vi "Main.vi"() -> ()   [LabVIEW 2017]
doc: "The myRIO Project template acquires acceleration data from the onboard accelerometer and displays the changes of acceleration values in a waveform chart."
uses:
  StateMachineControl.ctl
  <vilib>/Platform/TimedLoop/XDataNode/timing_clust.ctl
  <vilib>/Platform/TimedLoop/XDataNode/nitl_modes.ctl
  <vilib>/Platform/TimedLoop/XDataNode/wakeup.ctl
  <vilib>/myRIO/Instrument Drivers/Onboard IO/DIO/typedefs/DIO Reference.ctl
  <vilib>/myRIO/Common/Instrument Driver Framework/Utilities/typedefs/myRIO Generic Hardware Reference.ctl
  <vilib>/myRIO/Common/Instrument Driver Framework/Utilities/typedefs/Hardware Version Enum.ctl
  <vilib>/myRIO/Common/Instrument Driver Framework/Utilities/typedefs/myRIO v1.0 Reference.ctl
  <vilib>/myRIO/Common/Instrument Driver Framework/Utilities/typedefs/Generic FPGA Reference.ctl
  <vilib>/myRIO/Common/Instrument Driver Framework/myRIO v1.0/DIO/typedefs/DIO Channels List.ctl
  <vilib>/myRIO/Common/Instrument Driver Framework/myRIO v1.0/DIO/typedefs/DIO Channels Enum.ctl
  <vilib>/userdefined/High Color/nirio_resource_hc.ctl
  <vilib>/myRIO/Common/Instrument Driver Framework/myRIO v1.0/Encoder/typedefs/Encoder Signal Mode.ctl
  <vilib>/myRIO/Instrument Drivers/Onboard IO/Encoder/typedefs/Encoder Reference.ctl
  <vilib>/myRIO/Common/Instrument Driver Framework/myRIO v1.0/Encoder/typedefs/Encoder Channels Enum.ctl
  <vilib>/myRIO/Common/Instrument Driver Framework/myRIO v1.0/Encoder/typedefs/Encoder Configuration v1.0.ctl
  <vilib>/myRIO/Instrument Drivers/Onboard IO/PWM/typedefs/PWM Reference.ctl
  <vilib>/myRIO/Common/Instrument Driver Framework/myRIO v1.0/PWM/typedefs/PWM Channels Enum.ctl
  <vilib>/myRIO/Instrument Drivers/Onboard IO/PWM/typedefs/PWM Configuration.ctl
  <vilib>/myRIO/Common/Instrument Driver Framework/Utilities/vis/Is FPGA Ref Available.vi
  <vilib>/myRIO/Common/Instrument Driver Framework/myRIO v1.0/DIO/vis/myRIO v1.1 Open DIO.vi
  <vilib>/myRIO/Instrument Drivers/Onboard IO/DIO/vis/Read.vi
  <vilib>/myRIO/Instrument Drivers/Onboard IO/DIO/vis/Write.vi
  <vilib>/myRIO/Common/Instrument Driver Framework/myRIO v1.0/Encoder/vis/myRIO v1.1 Open Encoder.vi
  <vilib>/myRIO/Instrument Drivers/Onboard IO/Encoder/vis/Read.vi
  <vilib>/myRIO/Common/Instrument Driver Framework/myRIO v1.0/PWM/vis/myRIO v1.1 Open PWM.vi
  <vilib>/myRIO/Instrument Drivers/Onboard IO/PWM/vis/Set Duty Cycle and Frequency.vi
  <vilib>/myRIO/Common/Instrument Driver Framework/Utilities/vis/Validate Channels.vi
  <vilib>/myRIO/Common/Instrument Driver Framework/myRIO v1.0/DIO/vis/myRIO v1.0 Reserve DIO.vi
  <vilib>/myRIO/Common/Instrument Driver Framework/myRIO v1.0/Encoder/vis/myRIO v1.0 Reserve Encoder.vi
  <vilib>/myRIO/Common/Instrument Driver Framework/myRIO v1.0/PWM/vis/myRIO v1.0 Reserve PWM.vi
  <vilib>/myRIO/Common/Instrument Driver Framework/myRIO v1.0/UART/vis/myRIO v1.0 Close UART.vi
  <vilib>/myRIO/Common/Instrument Driver Framework/myRIO v1.0/Resource Manager/vis/myRIO v1.0 Reserve Channel List.vi
  <vilib>/myRIO/Common/Instrument Driver Framework/myRIO v1.0/DIO/vis/myRIO v1.0 Build MUX Configuration DIO.vi
  <vilib>/myRIO/Common/Instrument Driver Framework/myRIO v1.0/Encoder/vis/myRIO v1.0 Build MUX Configuration Encoder.vi
  <vilib>/myRIO/Common/Instrument Driver Framework/myRIO v1.0/PWM/vis/myRIO v1.0 Build MUX Configuration PWM.vi
  <vilib>/myRIO/Common/Instrument Driver Framework/myRIO v1.0/Resource Manager/vis/myRIO v1.0 Reserve Channel.vi
  <vilib>/myRIO/Common/Instrument Driver Framework/myRIO v1.0/Resource Manager/vis/myRIO v1.0 Unreserve Channel.vi
  <vilib>/myRIO/Common/Instrument Driver Framework/myRIO v1.0/Resource Manager/vis/myRIO v1.0 Create Configuration List.vi
  <vilib>/myRIO/Common/Instrument Driver Framework/myRIO v1.0/Resource Manager/vis/myRIO v1.0 Build Mutex Name.vi
  <vilib>/Utility/VariantDataType/GetNumericInfo.vi
  <vilib>/Utility/error.llb/Error Cluster From Error Code.vi
  <vilib>/myRIO/Common/Instrument Driver Framework/myRIO v1.0/myRIO v1.1 Open.vi
  <vilib>/myRIO/Common/Instrument Driver Framework/Utilities/vis/IO Manager.vi
  <vilib>/myRIO/Common/Instrument Driver Framework/Utilities/vis/Configuration Manager.vi
  <vilib>/myRIO/Common/Instrument Driver Framework/myRIO v1.0/Resource Manager/vis/myRIO v1.0 Configure IO.vi
  <vilib>/myRIO/Common/Instrument Driver Framework/myRIO v1.0/myRIO v1.0 Close.vi
  <vilib>/myRIO/Common/Instrument Driver Framework/myRIO v1.0/DIO/vis/myRIO v1.0 Read DIO.vi
  <vilib>/myRIO/Common/Instrument Driver Framework/myRIO v1.0/DIO/vis/myRIO v1.0 Write DIO.vi
  <vilib>/myRIO/Common/Instrument Driver Framework/myRIO v1.0/Encoder/vis/myRIO v1.0 Configure Encoder.vi
  <vilib>/myRIO/Common/Instrument Driver Framework/myRIO v1.0/Encoder/vis/myRIO v1.0 Read Encoder.vi
  <vilib>/myRIO/Common/Instrument Driver Framework/myRIO v1.0/PWM/vis/myRIO v1.0 Write PWM.vi
  <vilib>/myRIO/Common/Instrument Driver Framework/Utilities/vis/FPGA Ref Manager.vi
  <vilib>/myRIO/Common/Instrument Driver Framework/myRIO v1.0/myRIO v1.0 Reset FPGA.vi
  <vilib>/myRIO/Common/Instrument Driver Framework/myRIO v1.0/IRQ/vis/myRIO v1.0 IRQ Info FGV.vi
  <vilib>/myRIO/Common/Instrument Driver Framework/myRIO v1.0/IRQ/vis/myRIO v1.0 Timer IRQ Info FGV.vi
  <vilib>/myRIO/Common/Instrument Driver Framework/myRIO v1.0/IRQ/vis/myRIO v1.0 ISR Agent.vi
  <vilib>/Platform/TimedLoop/XDataNode/XDataNode.xnode
  <vilib>/myRIO/Express VI/Onboard Devices/Button/Button Express VI.xnode
  <vilib>/myRIO/Instrument Drivers/Onboard IO/DIO/vis/myRIO DIO Open.xnode
  <vilib>/myRIO/Express VI/Onboard Devices/LED/LED Express VI.xnode
  <vilib>/myRIO/Express VI/Onboard IO/Encoder/Encoder Express VI.xnode
  <vilib>/myRIO/Common/Instrument Driver Framework/myRIO v1.0/Encoder/typedefs/Encoder Count Direction Enum.ctl
  <vilib>/myRIO/Instrument Drivers/Onboard IO/Encoder/vis/myRIO Encoder Open.xnode
  <vilib>/myRIO/Express VI/Onboard IO/DO/DO Express VI.xnode
  <vilib>/myRIO/Express VI/Onboard IO/PWM/PWM Express VI.xnode
  <vilib>/myRIO/Instrument Drivers/Onboard IO/PWM/vis/myRIO PWM Open.xnode
  <vilib>/myRIO/Instrument Drivers/Utilities/Utilities.lvlib
  <vilib>/myRIO/Instrument Drivers/Onboard IO/Encoder/Encoder.lvlib
  <vilib>/myRIO/Instrument Drivers/Onboard IO/DIO/DIO.lvlib
  <vilib>/myRIO/Instrument Drivers/Onboard IO/PWM/PWM.lvlib
  <vilib>/Platform/TimedLoop/XDataNode/XDNodeRunTimeDep.lvlib
panel:
  in  "Marked Heading":dbl
  in  "Marked Distance":dbl
  in  "Go!":bool
  in  "Robot Heading":dbl
  out "Pixy Output Array":bool[](array[boolean])
  out "Detected":bool
  out "Data":string
  out "Color Signal Code":i32
  out "Object Actual Dist From Wall":dbl
  out "Object Y Average":dbl
  in  "Length":i32=90
  in  "Starting Index":i32
  out "Indexed Plot":cluster{dbl[], dbl[]}(graph)
  out "XY Graph":cluster{dbl[], dbl[]}(graph)
  in  "Robot Speed":dbl
  in  "Dist From Wall Setpoint":dbl=0.3
  out "LIDAR LOOP V_RIGHT":dbl
  out "LIDAR LOOP V_LEFT":dbl
  in  "Wall Tracking Boolean":bool
  out "Total Distance Travelled":dbl
  out "LIDAR Right x-avg (m)":dbl
  out "LIDAR Left x-avg (m)":dbl
  out "Min speed":dbl
  out "Max speed":dbl
  out "State":T1
  in  "Goal Position (m)":dbl[](array[numeric])=[2.0, 0.0]
  out "Theta Actual (rad)":dbl
  out "y":dbl
  out "x":dbl
  out "speed setpoint (m/s)":dbl
  out "chosen heading (rad)":dbl
  out "Output to PWM 2":dbl format="%.2f"
  out "Speed of Motor 2":dbl
  out "Motor 2 Total Distance":dbl
  out "Motor 2 Encoder Count":i32
  out "Counter Direction 2":enum16{"Counting Up", "Counting Down"}(ring)
  out "Overflow? 2":bool
  out "Motor 1 Total Distance":dbl
  out "Output to PWM":dbl format="%.2f"
  out "Speed of Motor 1":dbl
  out "Overflow?":bool
  out "Counter Direction":enum16{"Counting Up", "Counting Down"}(ring)
  out "Motor 1 Encoder Count":i32
  out "Error Out":errorcluster
  in  "Stop":bool
  # "Overview: This LabVIEW project is created to explore and analyse the data output provided by the encoder.\n\nAim of Encoder Data Analysis\n1. Process the number of counts generated by the encoder as the input.\n2. Output the motor speed and distance travelled."
  # "Motor 1"
  # "Motor 1 Encoder"
  # "Note: distance is in (m)"
  # "Note: speed is in (m/s)"
  # "Motor 2"
  # "Motor 2 Encoder"
  # "Note: speed is in (m/s)"
  # "Robot Control"
  # "Distance in m."
  # "Heading in (deg)."
  # "Speed is in m/s."
  # "Robot Position"
  # "Colour Sensor"
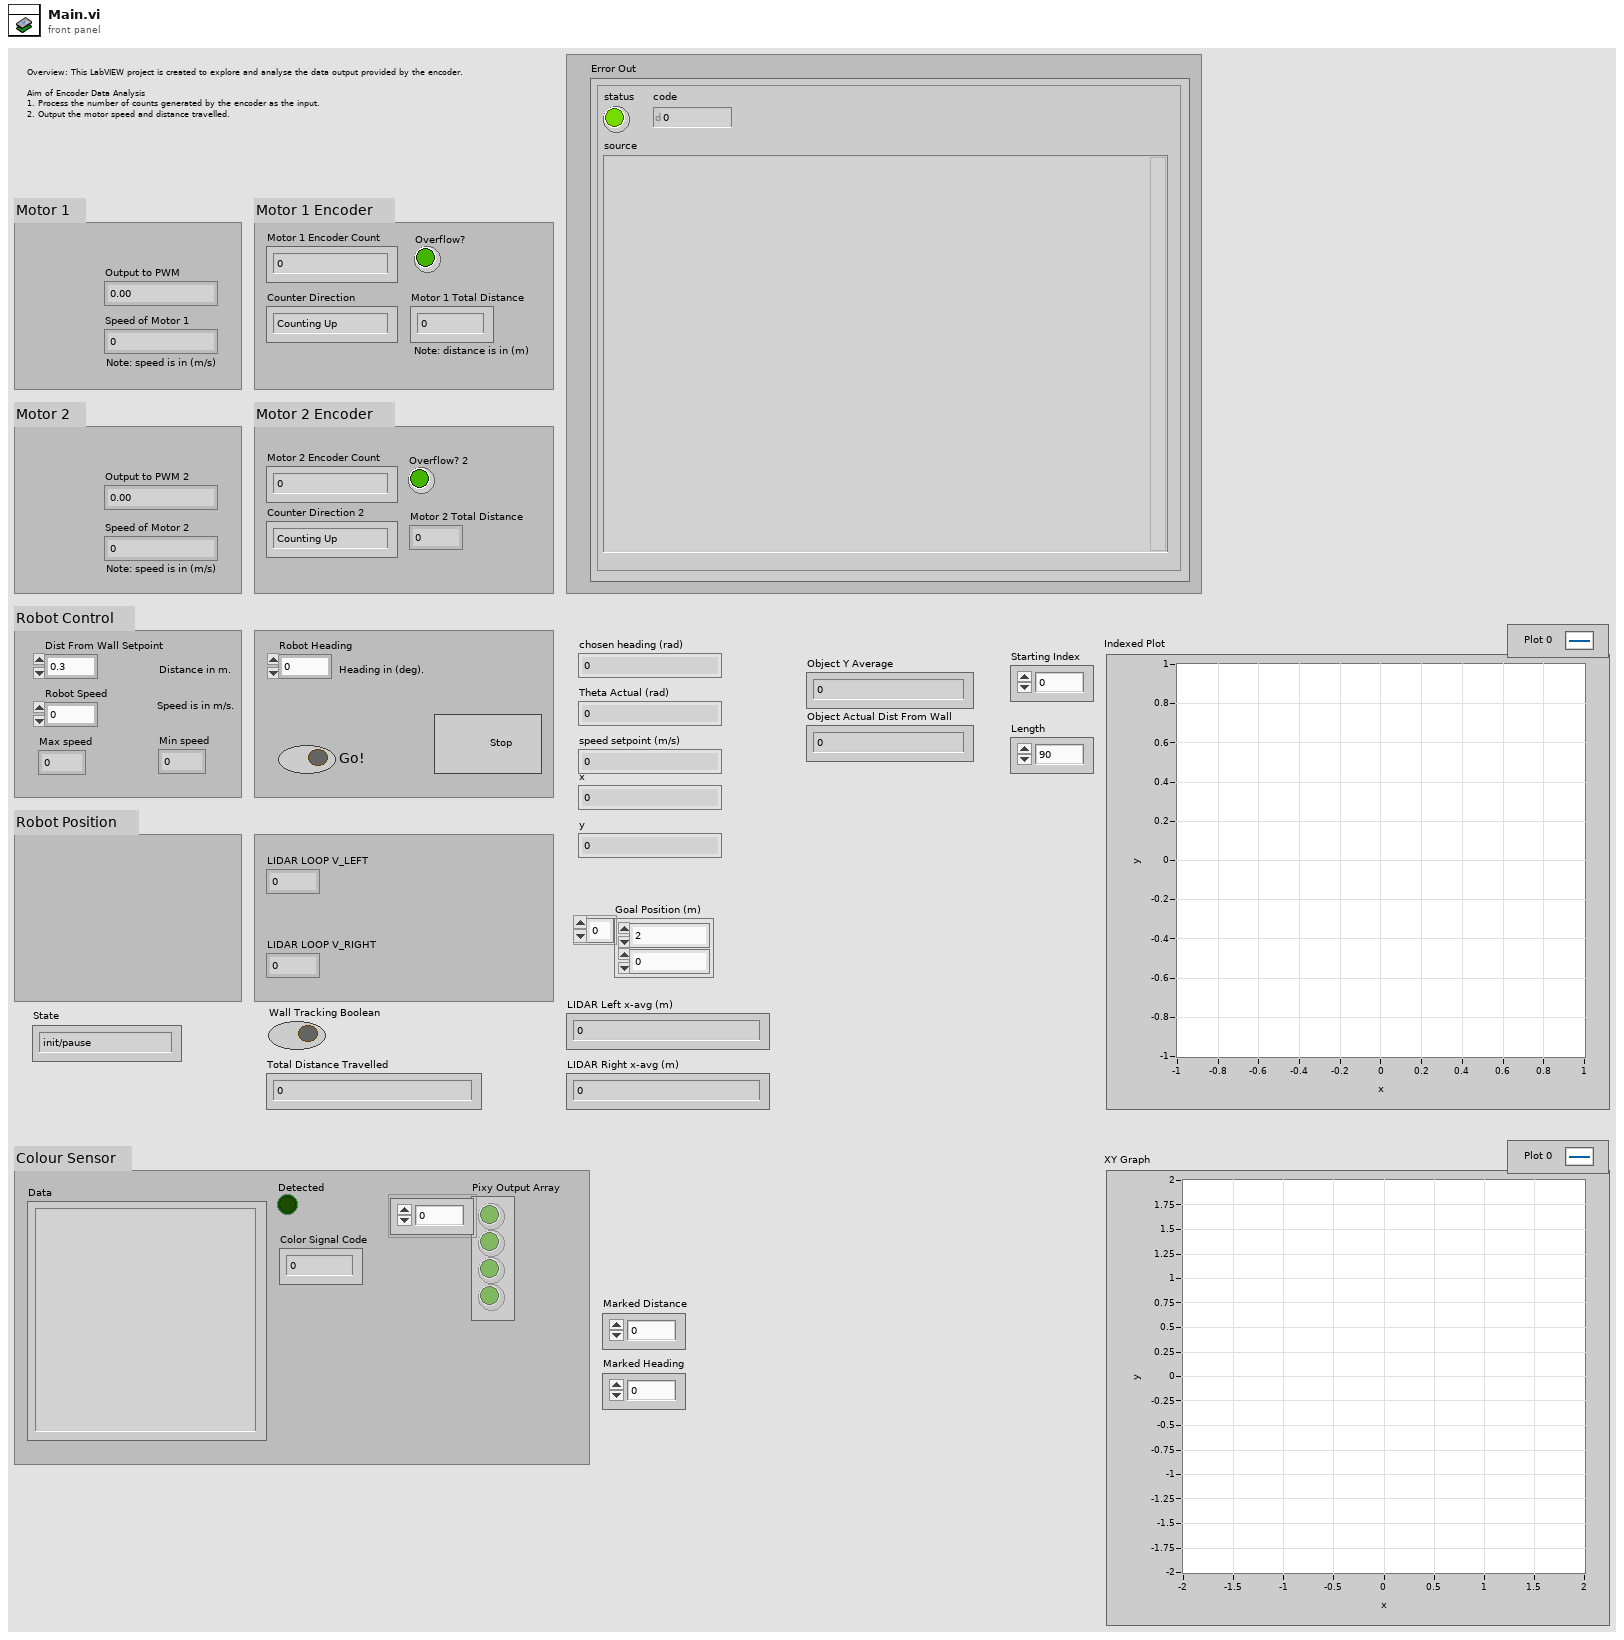
[diagram p1: front panel]
types:
  T1 = typedef "StateMachineControl.ctl" = enum16{"init/pause", "wall tracking w/ obs avoidance", "yellow zig-zag", "blue uneven surface", "red ramp", "green prepare to stop", "note down current distance", "go forward fixed dist & continue", "go forward fixed dist & stop", "stop finite state machine", "stop robot"}
  T2 = typedef "DIO.lvlib/DIO Reference.ctl" = cluster{"myRIO Reference":T3, "DIO Channels List":T7}
  T3 = typedef "myRIO Generic Hardware Reference.ctl" = cluster{"myRIO Model":T4, "myRIO Hardware Reference":T5}
  T4 = typedef "Hardware Version Enum.ctl" = enum16{"Unknown", "myRIO-1900", "myRIO-1950", "roboRIO", "NI ELVIS RIO CM"}
  T5 = typedef "myRIO v1.0 Reference.ctl" = cluster{"Generic FPGA Reference":T6, "Allow multiple opens":bool}
  T6 = typedef "Generic FPGA Reference.ctl" = refnum<k20>
  T7 = typedef "DIO Channels List.ctl" = T8[]
  T8 = typedef "DIO Channels Enum.ctl" = enum16{"Not Connected", "C/DIO0", "C/DIO1", "C/DIO2", "C/DIO3", "C/DIO4", "C/DIO5", "C/DIO6", "C/DIO7", "A/DIO0", "A/DIO1", "A/DIO2", "A/DIO3", "A/DIO4", "A/DIO5", "A/DIO6", "A/DIO7", "A/DIO8", "A/DIO9", "A/DIO10", "A/DIO11", "A/DIO12", "A/DIO13", "A/DIO14", "A/DIO15", "B/DIO0", "B/DIO1", "B/DIO2", "B/DIO3", "B/DIO4", "B/DIO5", "B/DIO6", "B/DIO7", "B/DIO8", "B/DIO9", "B/DIO10", "B/DIO11", "B/DIO12", "B/DIO13", "B/DIO14", "B/DIO15", "LED0", "LED1", "LED2", "LED3", "Button0", "DIO/DIO0", "DIO/DIO1", "DIO/DIO2", "DIO/DIO3", "DIO/DIO4", "DIO/DIO5", "DIO/DIO6", "DIO/DIO7", "DIO/DIO8", "DIO/DIO9", "SPI/CS0", "SPI/CS1", "SPI/CS2", "SPI/CS3", "LED RADIO (Green)", "LED RADIO (Red)", "LED COMM (Green)", "LED COMM (Red)", "LED MODE (Green)", "LED MODE (Red)"}
  T9 = typedef "nirio_resource_hc.ctl" = tag
  T10 = typedef "XDNodeRunTimeDep.lvlib/timing_clust.ctl" = cluster{"Expected End [f-1]":u64, "Actual End [f-1]":u64, "Finished Late? [f-1]":bool, "Expected End [i-1]":u64, "Actual End [i-1]":u64, "Finished Late? [i-1]":bool, "Expected Start [i]":u64, "Actual Start [i]":u64, "Expected Start [f]":u64, "Actual Start [f]":u64, "Source Name":string, "Structure Name":string, "Period":i64, "Deadline":i64, "Offset":i64, "Start":i64, "Priority":i32, "Timeout":i32, "Mode":T11, "Wakeup Reason":T12, "Error":errorcluster, "Source Type":string, "Secondary Source Type":string, "Global End Time":u64, "Global Start Time":u64, "Frame Duration":u64, "Iteration Duration":u64, "Assigned CPU":i32, "I/O Scan Engine Mode":u32}
  T11 = typedef "XDNodeRunTimeDep.lvlib/nitl_modes.ctl" = enum32{"No Change", "Process missed periods, maintain original phase", "Discard missed periods, maintain original phase", "Process missed periods, ignore original phase", "Discard missed periods, ignore original phase"}
  T12 = typedef "XDNodeRunTimeDep.lvlib/wakeup.ctl" = enum32{"Normal", "Aborted", "Asynchronous wakeup", "Timing source error", "Timed loop error", "Timeout"}
  T13 = typedef "PWM.lvlib/PWM Reference.ctl" = cluster{"myRIO Reference":T3, "PWM Channels Enum":T14, "PWM Configuration":T15}
  T14 = typedef "PWM Channels Enum.ctl" = enum16{"Not Connected", "C/PWM0", "C/PWM1", "A/PWM0", "A/PWM1", "A/PWM2", "B/PWM0", "B/PWM1", "B/PWM2", "PWM/PWM0", "PWM/PWM1", "PWM/PWM2", "PWM/PWM3", "PWM/PWM4", "PWM/PWM5", "PWM/PWM6", "PWM/PWM7", "PWM/PWM8", "PWM/PWM9"}
  T15 = typedef "PWM.lvlib/PWM Configuration.ctl" = cluster{"Frequency":dbl, "Duty Cycle":dbl}
  T16 = typedef "Encoder.lvlib/Encoder Reference.ctl" = cluster{"myRIO Reference":T3, "Encoder Channels Enum":T17}
  T17 = typedef "Encoder Channels Enum.ctl" = enum16{"Not Connected", "C/ENC0", "C/ENC1", "A/ENC", "B/ENC", "DIO/ENC0", "DIO/ENC1", "DIO/ENC2", "DIO/ENC3", "DIO/ENC4"}
  T18 = typedef "Encoder Signal Mode.ctl" = enum16{"Quadrature phase signal", "Step and direction signal"}
  T19 = typedef "Encoder Count Direction Enum.ctl" = enum16{"Counting Up", "Counting Down"}
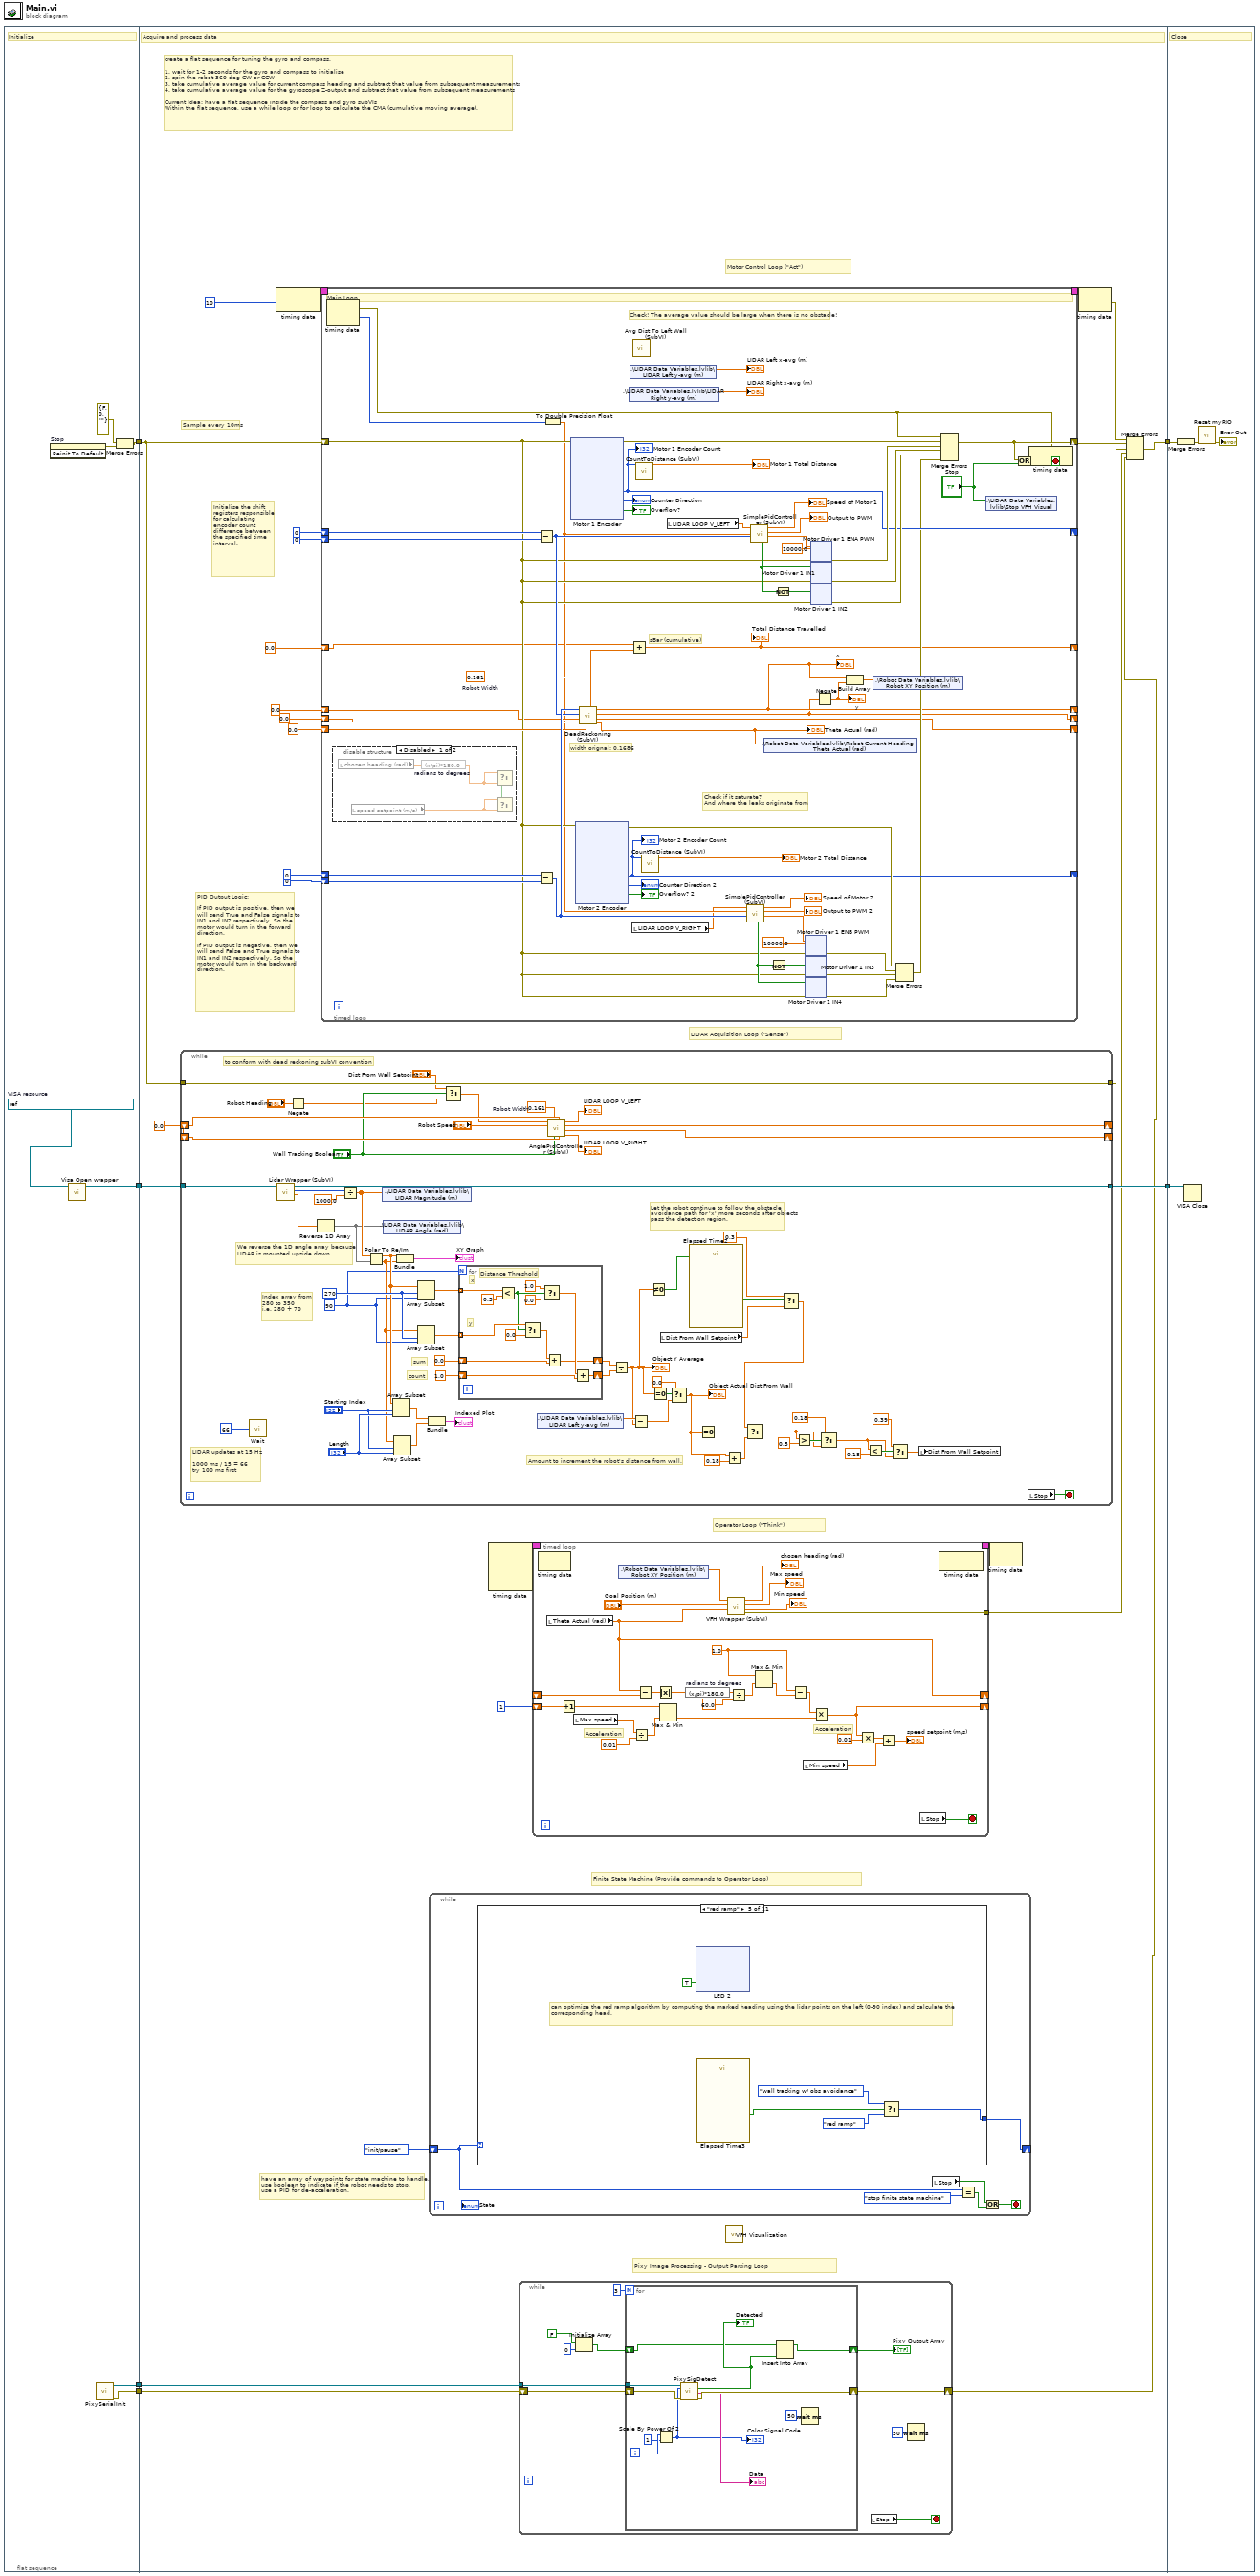
[diagram p0: block diagram]
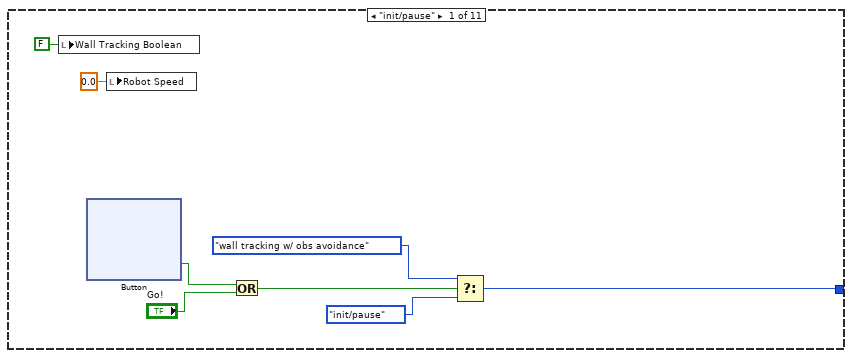
[diagram p2: hidden frame]
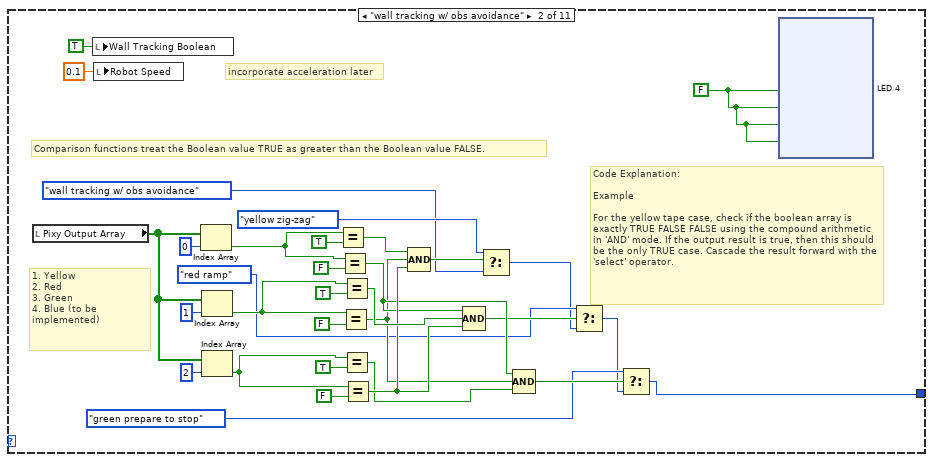
[diagram p3: hidden frame]
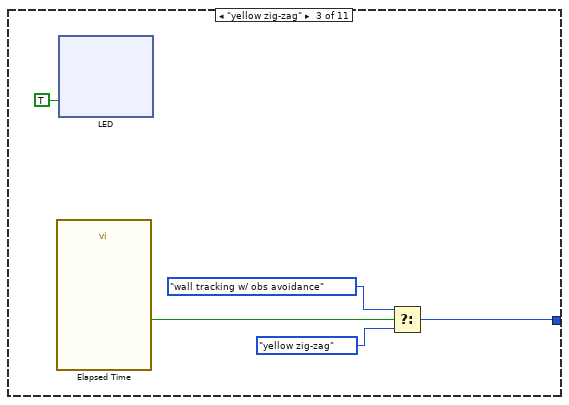
[diagram p4: hidden frame]
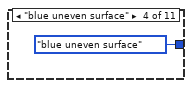
[diagram p5: hidden frame]
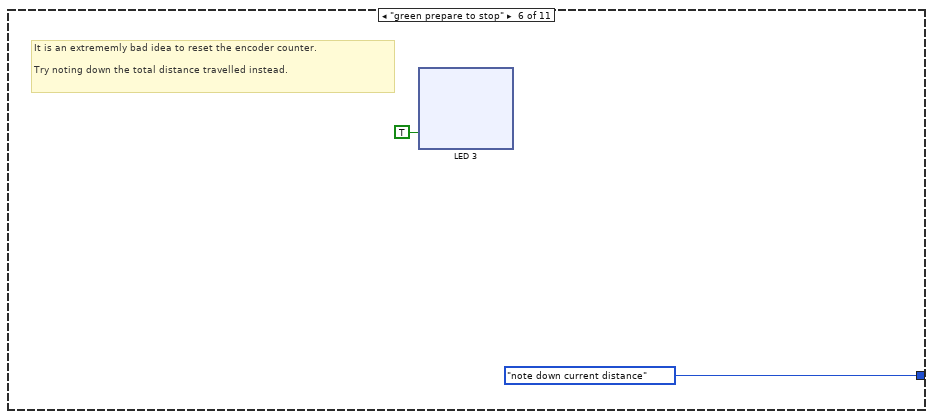
[diagram p6: hidden frame]
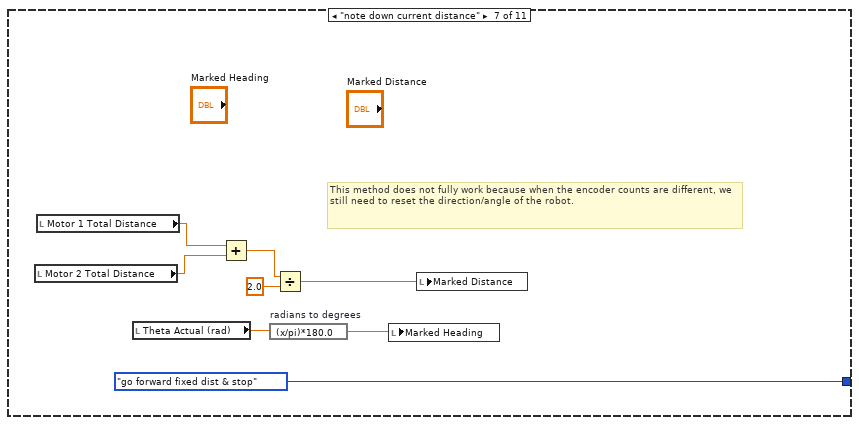
[diagram p7: hidden frame]
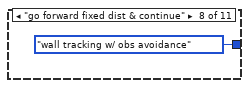
[diagram p8: hidden frame]
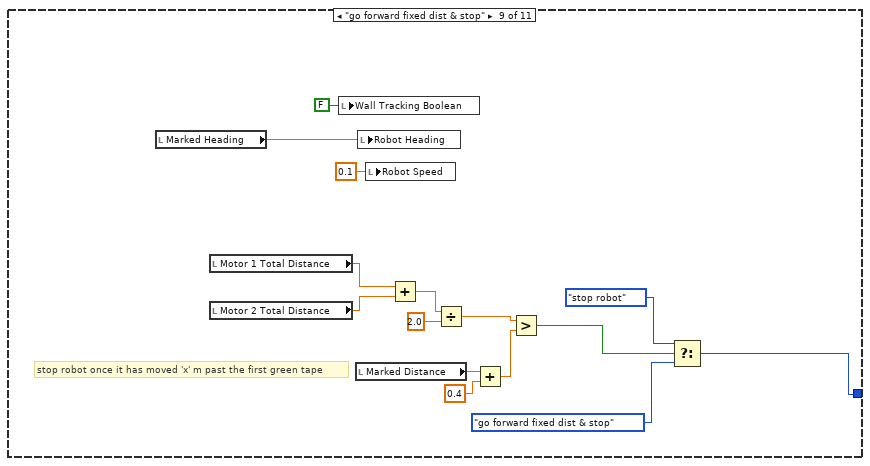
[diagram p9: hidden frame]
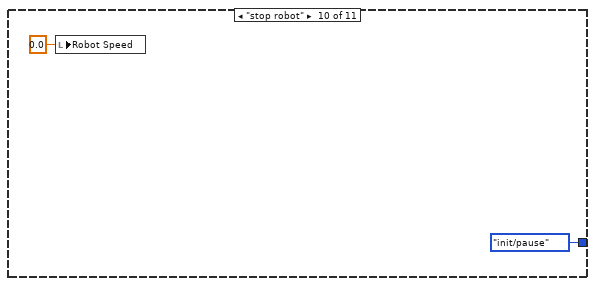
[diagram p10: hidden frame]
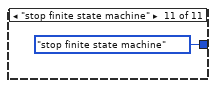
[diagram p11: hidden frame]
diagram:
  n1 = flat-sequence {
    tunnel: [w12] -> w6
    tunnel: [w10] -> w4
    tunnel: [w8] -> w2
    tunnel: [w7] -> w1
    tunnel: w6 -> [w26]
    tunnel: [w37] -> w5
    tunnel: w4 -> [w28]
    tunnel: [w27] -> w3
    tunnel: w2 -> [w16]
    tunnel: w1 -> [w15]
    tunnel: w5 -> [w810]
    tunnel: w3 -> [w811]
    frame #0 {
      w11 = refnum<visa-resource-name> "TCPIP::169.254.233.170::2112::SOCKET"  # VISA resource
      # "Initialize"
      n2 = invoke on="Stop" class="Bool (strict)" method="Reinit To Default"() -> (error out=w9:errorcluster)  [unwired: 3 in, 2 out]
      n3 = call "Visa Open wrapper.vi"("VISA resource"=w11) -> ("VISA resource name out"=w10:refnum<visa-resource-name>)  [unwired: 10 in]
      n4 = call "PixySerialInit.vi"() -> ("error out"=w7:errorcluster, "VISA resource name out"=w8:refnum<visa-resource-name>)  [unwired: 10 in]
      n5 = Merge Errors(errorcluster {"status"=FALSE, "code"=0, "source"=""} ("error in (no error)"), w9) -> (w12:errorcluster)
    }
    frame #1 {
      w18 = 0.0 ("Current Error")
      # "Pixy Image Processing - Output Parsing Loop"
      # "Finite State Machine (Provide commands to Operator Loop)"
      # "create a flat sequence for tuning the gyro and compass.\n\n1. wait for 1-2 seconds for the gyro and compass to initialise\n2. spin the robot 360 deg CW or CCW\n3. take cumulative average value for current compass heading and subtract that value from subsequent measurements\n4. take cumulative average value for the gyroscope Z-output and subtract that value from subsequent measurements\n\nCurrent Idea: have a flat sequence inside the compass and gyro subVIs\nWithin the flat sequence, use a while loop or for loop to calculate the CMA (cumulative moving average)."
      # "have an array of waypoints for state machine to handle,\nuse boolean to indicate if the robot needs to stop,\nuse a PID for de-acceleration."
      # "Operator Loop (\"Think\")"
      # "LIDAR Acquisition Loop (\"Sense\")"
      # "Motor Control Loop (\"Act\")"
      # "PID Output Logic:\n\nIf PID output is positive, then we will send True and False signals to IN1 and IN2 respectively. So the motor would turn in the forward direction.\n\nIf PID output is negative, then we will send False and True signals to IN1 and IN2 respectively. So the motor would turn in the backward direction."
      # "Initialise the shift registers responsible for calculating encoder count difference between the specified time interval."
      # "Sample every 10ms"
      # "Acquire and process data"
      n6 = while {
        tunnel: w28 -> [w419]
        tunnel: [w418] -> w27
        tunnel: w26 -> [w414]
        tunnel: [w414] -> w25
        shift-right: [w413] -> _
        shift-left: w18 -> [w411]
        shift-right: [w412] -> _
        shift-left: w18 -> [w410]
        stop <- w415 stop-if-true
        w392 = 90 ("length")
        w395 = 270 ("index")
        w407 = 0.161  # Robot Width
        # "to conform with dead reckoning subVI convention"
        # "Let the robot continue to follow the obstacle avoidance path for 'x' more seconds after objects pass the detection region."
        # "Amount to increment the robot's distance from wall."
        # "count"
        # "sum"
        # "Index array from 280 to 350\ni.e. 280 + 70"
        # "We reverse the 1D angle array because LIDAR is mounted upside down."
        # "LIDAR updates at 15 Hz\n\n1000 ms / 15 = 66\ntry 100 ms first"
        n7 = call "Wait"("Count(mSec)"=u32 66) -> ()  [unwired: 1 out]
        n8 = call "Lidar Wrapper (SubVI).vi"("VISA Refnum in"=w419) -> ("Array"=w401:dbl[], "Distance Array"=w400:u32[], "VISA Refnum out"=w418:refnum<visa-resource-name>)  [unwired: 8 in]
        n9 = Negate(x="Robot Heading") -> (-x=w358:dbl)
        n10 = Reverse 1D Array(array=w401) -> (reversed array=w396:dbl[])
        n11 = Divide(x=w400, y=1000.0) -> (x/y=w399:dbl[])
        n12 = Polar To Re/Im(2:w396, 3:w399) -> (0:w393:dbl[], 1:w394:dbl[])
        n13 = shared-variable ".\\LIDAR Data Variables.lvlib\\LIDAR Magnitude (m)"(w399) -> ()  [unwired: 1 in, 1 out]
        n14 = shared-variable ".\\LIDAR Data Variables.lvlib\\LIDAR Angle (rad)"(w396) -> ()  [unwired: 1 in, 1 out]
        n15 = Array Subset(array=w394, index="Starting Index", length="Length") -> (w403:dbl[])
        n16 = Array Subset(array=w393, index="Starting Index", length="Length") -> (w402:dbl[])
        n17 = Bundle(w394, w393) -> (→"XY Graph":cluster{dbl[], dbl[]})  [unwired: 1 in]
        n18 = Array Subset(array=w394, index=w395, length=w392) -> (w391:dbl[])
        n19 = Array Subset(array=w393, index=w395, length=w392) -> (w390:dbl[])
        n20 = Bundle(w403, w402) -> (→"Indexed Plot":cluster{dbl[], dbl[]})  [unwired: 1 in]
        n21 = Select(t="Dist From Wall Setpoint", s="Wall Tracking Boolean", f=w358) -> (s? t:f=w359:dbl)
        n22 = for {
          N: w392 -> [_]
          tunnel: w391 -> [w431] mode=indexing
          tunnel: w390 -> [w430] mode=indexing
          shift-right: [w421] -> w387
          shift-left: 0.0 ("y") -> [w427]
          shift-right: [w420] -> w386
          shift-left: 1.0 ("y") -> [w422]
          # "Distance Threshold"
          # "y"
          # "x"
          n23 = Less?(x=w431, y=0.3) -> (x < y?=w426:bool)
          n24 = Select(t=w430, s=w426, f=0.0) -> (s? t:f=w428:dbl)
          n25 = Select(t=1.0, s=w426, f=0.0) -> (s? t:f=w423:dbl)
          n26 = Add(x=w428, y=w427) -> (x+y=w421:dbl)
          n27 = Add(x=w423, y=w422) -> (x+y=w420:dbl)
        }
        n28 = shared-variable ".\\LIDAR Data Variables.lvlib\\LIDAR Left y-avg (m)"() -> (w385:dbl)  [unwired: 1 in, 1 out]
        n29 = call "AnglePidController (SubVI).vi"("Sum Error"=w410, "Previous Error"=w411, "Wall Tracking Boolean"="Wall Tracking Boolean", "Robot Width (m)"=w407, "Desired Speed (m|s)"="Robot Speed", "PID Setpoint [Wall Distance (m) OR Heading (deg)]"=w359) -> ("Velocity Right (m|s)"=→"LIDAR LOOP V_RIGHT":dbl, "Sum For Shift Register"=w412:dbl, "Current Error"=w413:dbl, "Velocity Left (m|s)"=→"LIDAR LOOP V_LEFT":dbl)  [unwired: 2 in]
        n30 = Divide(x=w387, y=w386) -> (x/y=w369:dbl)
        "Object Y Average" <- w369
        n31 = Subtract(x=w385, y=w369) -> (x-y=w370:dbl)
        n32 = Not Equal To 0?(x=w369) -> (x != 0?=w368:bool)
        n33 = Equal To 0?(x=w369) -> (x = 0?=w372:bool)
        n34 = local read "Dist From Wall Setpoint"() -> (w366:dbl)
        n35 = Select(t=0.0, s=w372, f=w370) -> (s? t:f=w363:dbl)
        "Object Actual Dist From Wall" <- w363
        n36 = call "Elapsed Time2"("Reset"=w368) -> ("Time has Elapsed"=w367:bool)  [unwired: 11 in, 7 out]
        n37 = Equal To 0?(x=w363) -> (x = 0?=w384:bool)
        n38 = Add(x=w363, y=0.18) -> (x+y=w382:dbl)
        n39 = Select(t=0.3, s=w367, f=w366) -> (s? t:f=w364:dbl)
        n40 = Select(t=w364, s=w384, f=w382) -> (s? t:f=w377:dbl)
        n41 = Greater?(x=w377, y=0.5) -> (0:w379:bool)
        n42 = Select(t=0.18, s=w379, f=w377) -> (s? t:f=w376:dbl)
        n43 = Less?(x=w376, y=0.18) -> (x < y?=w378:bool)
        n44 = Select(t=0.39, s=w378, f=w376) -> (s? t:f=w373:dbl)
        n45 = local write "Dist From Wall Setpoint"(w373) -> ()
        n46 = local read "Stop"() -> (w415:bool)
      }
      n47 = node-c288(i64 10 ("Period")) -> (w40:T10)
      n48 = timed-loop {
        shift-right: [w487] -> w35
        shift-left: w26 -> [w454]
        timing: w40 -> [_]
        timing-out: [_] -> w39
        shift-right: [w462] -> _
        shift-left: 0 ("Counter Value") -> [w466]
        shift-left: 0 ("Counter Value") -> [w464]
        shift-right: [w461] -> _
        shift-left: 0 ("Counter Value") -> [w465]
        shift-left: 0 ("Counter Value") -> [w463]
        shift-right: [w444] -> _
        shift-left: 0.0 ("x") -> [w449]
        shift-right: [w446] -> _
        shift-left: 0.0 ("Theta") -> [w458]
        shift-right: [w443] -> _
        shift-left: 0.0 ("y") -> [w448]
        shift-right: [w435] -> _
        shift-left: 0.0 -> [w436]
        stop <- w491 stop-if-true
        w450 = 0.161  # Robot Width
        # "Check if it saturate?\nAnd where the leaks originate from"
        # "Check! The average value should be large when there is no obstacle!"
        # "sBar (cumulative)"
        # "width orignal: 0.1686"
        # "Main Loop"
        n49 = node-c288() -> (w453:errorcluster, w482:i64)  [unwired: 1 in]
        n50 = disable-structure shown="Disabled" {
          frame Disabled {
            n51 = local read "chosen heading (rad)"() -> (w495:dbl)
            n52 = local read "speed setpoint (m/s)"() -> (w492:dbl)
            n53 = expression code="(x/pi)*180.0" "radians to degrees"(w495) -> (w493:dbl)
            n54 = Select(t=w493, f=w493) -> (s=w494:bool)  [unwired: 1 out]
            n55 = Select(t=w492, s=w494, f=w492) -> ()  [unwired: 1 out]
          }
          frame Enabled {
          }
        }
        n56 = Subtract(x=w466, y=w464) -> (x-y=w459:i32)
        n57 = Subtract(x=w465, y=w463) -> (x-y=w460:i32)
        n58 = To Double Precision Float(number=w482) -> (double precision float=w440:dbl)
        n59 = xnode "Motor 1 Encoder"("error in (no error)"=w454) -> ("Counter Value"=w462:i32, "Counter Direction"=→"Counter Direction":T19, "Overflow?"=→"Overflow?":bool, "error out"=w488:errorcluster)  [unwired: 1 in]
        "Motor 1 Encoder Count" <- w462
        n60 = xnode ("Motor 2 Encoder")("error in (no error)"=w454) -> ("Counter Value"=w461:i32, "Counter Direction"=→"Counter Direction 2":T19, "Overflow?"=→"Overflow? 2":bool, "error out"=w471:errorcluster)  [unwired: 1 in]
        "Motor 2 Encoder Count" <- w461
        n61 = call "DeadReckoning (SubVI).vi"("Theta_0"=w458, "Robot Width"=w450, "y0"=w448, "x0"=w449, "sL"=w459, "sR"=w460) -> ("Theta Actual (rad)"=w445:dbl, "Theta (rad)"=w446:dbl, "y"=w443:dbl, "x"=w444:dbl, "sBar"=w437:dbl)  [unwired: 1 in]
        "x" <- w444
        "Theta Actual (rad)" <- w445
        n62 = shared-variable ".\\LIDAR Data Variables.lvlib\\LIDAR Right y-avg (m)"() -> (→"LIDAR Right x-avg (m)":dbl)  [unwired: 1 in, 1 out]
        n63 = shared-variable ".\\LIDAR Data Variables.lvlib\\LIDAR Left y-avg (m)"() -> (→"LIDAR Left x-avg (m)":dbl)  [unwired: 1 in, 1 out]
        n64 = Add(x=w436, y=w437) -> (x+y=w435:dbl)
        "Total Distance Travelled" <- w435
        n65 = local read "LIDAR LOOP V_RIGHT"() -> (w433:dbl)
        n66 = call "Avg Dist To Left Wall (SubVI).vi"() -> ()  [unwired: 12 in]
        n67 = call "CountToDistance (SubVI).vi"("Counter Value"=w462) -> ("Total Distance Travelled (m)"=→"Motor 1 Total Distance":dbl)  [unwired: 10 in]
        n68 = call "CountToDistance (SubVI).vi"("Counter Value"=w461) -> ("Total Distance Travelled (m)"=→"Motor 2 Total Distance":dbl)  [unwired: 10 in]
        n69 = local read "LIDAR LOOP V_LEFT"() -> (w434:dbl)
        n70 = call "SimplePidController (SubVI).vi"("Encoder Count Difference"=w460, "Period of Timed Loop"=w440, "Speed Setpoint"=w433) -> ("Output to Duty Cycle"=w456:dbl, "Output to PWM"=→"Output to PWM 2":dbl, "Speed of Motor"=→"Speed of Motor 2":dbl, "Boolean Output for Motor Driver"=w467:bool)  [unwired: 5 in]
        n71 = call "SimplePidController (SubVI).vi"("Encoder Count Difference"=w459, "Period of Timed Loop"=w440, "Speed Setpoint"=w434) -> ("Output to Duty Cycle"=w457:dbl, "Output to PWM"=→"Output to PWM":dbl, "Speed of Motor"=→"Speed of Motor 1":dbl, "Boolean Output for Motor Driver"=w470:bool)  [unwired: 5 in]
        n72 = shared-variable ".\\Robot Data Variables.lvlib\\Robot Current Heading - Theta Actual (rad)"(w445) -> ()  [unwired: 1 in, 1 out]
        n73 = Not(x=w467) -> (.not. x?=w468:bool)
        n74 = Not(x=w470) -> (.not. x?=w469:bool)
        n75 = xnode "Motor Driver 1 ENB PWM"("error in (no error)"=w454, "Duty Cycle"=w456, "Frequency [Hz]"=10000.0) -> ("error out"=w476:errorcluster)
        n76 = xnode "Motor Driver 1 IN3"("error in (no error)"=w454, "A/DIO2 (Pin 15)"=w468) -> ("error out"=w475:errorcluster)
        n77 = xnode "Motor Driver 1 IN4"("error in (no error)"=w454, "A/DIO3 (Pin 17)"=w467) -> ("error out"=w474:errorcluster)
        n78 = xnode "Motor Driver 1 ENA PWM"("error in (no error)"=w454, "Duty Cycle"=w457, "Frequency [Hz]"=10000.0) -> ("error out"=w483:errorcluster)
        n79 = xnode "Motor Driver 1 IN1"("error in (no error)"=w454, "A/DIO0 (Pin 11)"=w470) -> ("error out"=w486:errorcluster)
        n80 = xnode "Motor Driver 1 IN2"("error in (no error)"=w454, "A/DIO1 (Pin 13)"=w469) -> ("error out"=w485:errorcluster)
        n81 = Negate(x=w443) -> (-x=w441:dbl)
        "y" <- w441
        n82 = Build Array(w444, w441) -> (w442:dbl[])
        n83 = shared-variable ".\\Robot Data Variables.lvlib\\Robot XY Position (m)"(w442) -> ()  [unwired: 1 in, 1 out]
        n84 = Merge Errors(w471, w476, w475, w474) -> (w455:errorcluster)
        n85 = Merge Errors "Merge Errors"(w453, w488, w483, w486, w485, w455) -> (w487:errorcluster)
        n86 = shared-variable ".\\LIDAR Data Variables.lvlib\\Stop VFH Visual"("Stop") -> ()  [unwired: 1 in, 1 out]
        n87 = Or(x=w487, y="Stop") -> (x .or. y?=w491:bool)
        n88 = node-c288(w453) -> ()  [unwired: 1 out]
      }
      n89 = while {
        shift-right: [w65] -> _
        shift-left: StateMachineControl."init/pause" ("State") -> [w67]
        stop <- w63 stop-if-true
        n90 = case shown="\"red ramp\"" w67 {
          tunnel: [w72 w112 w182 StateMachineControl."blue uneven surface" ("State") w223 StateMachineControl."note down current distance" ("State") StateMachineControl."go forward fixed dist & stop" ("State") StateMachineControl."wall tracking w/ obs avoidance" ("State") w312 StateMachineControl."init/pause" ("State") StateMachineControl."stop finite state machine" ("State")] -> w65
          frame "init/pause" {
            n91 = local write "Wall Tracking Boolean"(FALSE ("Wall Tracking Boolean")) -> ()
            n92 = xnode "Button"() -> ("Value"=w71:bool)  [unwired: 1 in, 1 out]
            n93 = local write "Robot Speed"(0.0 ("Robot Speed")) -> ()
            n94 = Or(x=w71, y="Go!") -> (x .or. y?=w69:bool)
            n95 = Select(t=StateMachineControl."wall tracking w/ obs avoidance" ("State"), s=w69, f=StateMachineControl."init/pause" ("State")) -> (s? t:f=w72:T1)
          }
          frame "wall tracking w/ obs avoidance" {
            w111 = FALSE ("LED0")
            # "Code Explanation:\n\nExample\n\nFor the yellow tape case, check if the boolean array is exactly TRUE FALSE FALSE using the compound arithmetic in 'AND' mode. If the output result is true, then this should be the only TRUE case. Cascade the result forward with the 'select' operator."
            # "Comparison functions treat the Boolean value TRUE as greater than the Boolean value FALSE."
            # "1. Yellow\n2. Red\n3. Green\n4. Blue (to be implemented)"
            # "incorporate acceleration later"
            n96 = local read "Pixy Output Array"() -> (w137:bool[])
            n97 = local write "Wall Tracking Boolean"(TRUE ("Wall Tracking Boolean")) -> ()
            n98 = local write "Robot Speed"(0.1 ("Robot Speed")) -> ()
            n99 = Index Array(array=w137, index=0) -> (element=w125:bool)
            n100 = Index Array(array=w137, index=1) -> (element=w124:bool)
            n101 = Index Array(array=w137, index=2) -> (element=w126:bool)
            n102 = Equal?(x=w125, y=TRUE) -> (x = y?=w133:bool)
            n103 = Equal?(x=w125, y=FALSE) -> (x = y?=w121:bool)
            n104 = Equal?(x=w124, y=FALSE) -> (x = y?=w120:bool)
            n105 = Equal?(x=w124, y=TRUE) -> (x = y?=w123:bool)
            n106 = Equal?(x=w126, y=TRUE) -> (x = y?=w119:bool)
            n107 = Equal?(x=w126, y=FALSE) -> (x = y?=w122:bool)
            n108 = Compound Arithmetic op=AND(w133, w120, w122) -> (w132:bool)
            n109 = Compound Arithmetic op=AND(w121, w123, w122) -> (w118:bool)
            n110 = Select(t=StateMachineControl."yellow zig-zag" ("State"), s=w132, f=StateMachineControl."wall tracking w/ obs avoidance" ("State")) -> (s? t:f=w116:T1)
            n111 = Compound Arithmetic op=AND(w121, w120, w119) -> (w115:bool)
            n112 = Select(t=StateMachineControl."red ramp" ("State"), s=w118, f=w116) -> (s? t:f=w113:T1)
            n113 = Select(t=StateMachineControl."green prepare to stop" ("State"), s=w115, f=w113) -> (s? t:f=w112:T1)
            n114 = xnode "LED 4"("LED0"=w111, "LED1"=w111, "LED2"=w111, "LED3"=w111) -> ()  [unwired: 1 in, 1 out]
          }
          frame "yellow zig-zag" {
            n115 = call "Elapsed Time"() -> ("Time has Elapsed"=w185:bool)  [unwired: 12 in, 7 out]
            n116 = xnode "LED"("LED0"=TRUE) -> ()  [unwired: 1 in, 1 out]
            n117 = Select(t=StateMachineControl."wall tracking w/ obs avoidance" ("State"), s=w185, f=StateMachineControl."yellow zig-zag" ("State")) -> (s? t:f=w182:T1)
          }
          frame "blue uneven surface" {
          }
          frame "red ramp" {
            # "can optimise the red ramp algorithm by computing the marked heading using the lidar points on the left (0-90 index) and calculate the corresponding head."
            n118 = xnode "LED 2"("LED1"=TRUE) -> ()  [unwired: 1 in, 1 out]
            n119 = call "Elapsed Time3"() -> ("Time has Elapsed"=w226:bool)  [unwired: 12 in, 7 out]
            n120 = Select(t=StateMachineControl."wall tracking w/ obs avoidance" ("State"), s=w226, f=StateMachineControl."red ramp" ("State")) -> (s? t:f=w223:T1)
          }
          frame "green prepare to stop" {
            # "It is an extrememly bad idea to reset the encoder counter.\n\nTry noting down the total distance travelled instead."
            n121 = xnode "LED 3"("LED2"=TRUE) -> ()  [unwired: 1 in, 1 out]
          }
          frame "note down current distance" {
            # "This method does not fully work because when the encoder counts are different, we still need to reset the direction/angle of the robot."
            n122 = local read "Motor 2 Total Distance"() -> (w304:dbl)
            n123 = local read "Motor 1 Total Distance"() -> (w305:dbl)
            n124 = local read "Theta Actual (rad)"() -> (w300:dbl)
            n125 = Add(x=w305, y=w304) -> (x+y=w302:dbl)
            n126 = expression code="(x/pi)*180.0" "radians to degrees"(w300) -> (w299:dbl)
            n127 = Divide(x=w302, y=2.0) -> (x/y=w301:dbl)
            n128 = local write "Marked Heading"(w299) -> ()
            n129 = local write "Marked Distance"(w301) -> ()
          }
          frame "go forward fixed dist & continue" {
          }
          frame "go forward fixed dist & stop" {
            # "stop robot once it has moved 'x' m past the first green tape"
            n130 = local read "Marked Heading"() -> (w308:dbl)
            n131 = local read "Motor 1 Total Distance"() -> (w320:dbl)
            n132 = local read "Motor 2 Total Distance"() -> (w319:dbl)
            n133 = local write "Wall Tracking Boolean"(FALSE ("Wall Tracking Boolean")) -> ()
            n134 = local read "Marked Distance"() -> (w310:dbl)
            n135 = local write "Robot Heading"(w308) -> ()
            n136 = local write "Robot Speed"(0.1 ("Robot Speed")) -> ()
            n137 = Add(x=w320, y=w319) -> (x+y=w318:dbl)
            n138 = Divide(x=w318, y=2.0) -> (x/y=w316:dbl)
            n139 = Add(x=w310, y=0.4) -> (x+y=w309:dbl)
            n140 = Greater?(x=w316, y=w309) -> (0:w315:bool)
            n141 = Select(t=StateMachineControl."stop robot" ("State"), s=w315, f=StateMachineControl."go forward fixed dist & stop" ("State")) -> (s? t:f=w312:T1)
          }
          frame "stop robot" {
            n142 = local write "Robot Speed"(0.0 ("Robot Speed")) -> ()
          }
          frame "stop finite state machine" {
          }
        }
        n143 = local read "Stop"() -> (w62:bool)
        n144 = Equal?(x=w67, y=StateMachineControl."stop finite state machine") -> (x = y?=w64:bool)
        n145 = Or(x=w62, y=w64) -> (x .or. y?=w63:bool)
      }
      n146 = node-c288() -> (w24:T10)  [unwired: 4 in]
      n147 = while {
        shift-right: [w50] -> w14
        shift-left: w15 -> [w43]
        tunnel: w16 -> [w42]
        stop <- w41 stop-if-true
        n148 = Initialize Array(FALSE, 0 ("dimension size")) -> (w46:bool[])
        n149 = for {
          N: 3 -> [_]
          tunnel: w42 -> [w61]
          shift-right: [w59] -> w50
          shift-left: w43 -> [w60]
          shift-right: [w55] -> w47
          shift-left: w46 -> [w54]
          i -> [w52]
          n150 = Scale By Power Of 2(n=w52, x=u8 1) -> (x*2^n=w53:u8)
          "Color Signal Code" <- w53
          n151 = call "PixySigDetect.vi"("error in (no error)"=w60, "Signature Number"=w53, "VISA resource name"=w61) -> ("error out"=w59:errorcluster, "Data"=→"Data":string, "Detected"=w56:bool)  [unwired: 5 in, 1 out]
          "Detected" <- w56
          n152 = Insert Into Array(array=w54, new element=w56) -> (w55:bool[])  [unwired: 1 in]
          n153 = Wait (ms)(milliseconds to wait=u32 50) -> ()  [unwired: 1 out]
        }
        "Pixy Output Array" <- w47
        n154 = local read "Stop"() -> (w41:bool)
        n155 = Wait (ms)(milliseconds to wait=u32 50) -> ()  [unwired: 1 out]
      }
      n156 = timed-loop {
        timing: w24 -> [_]
        timing-out: [_] -> w23
        tunnel: [w351] -> w21
        shift-right: [w344] -> _
        shift-left: 1 -> [w349]
        shift-right: [w339] -> _
        shift-left: _ -> [w348]
        stop <- w353 stop-if-true
        w331 = 1.0 ("y")
        # "Acceleration"
        # "Acceleration"
        n157 = node-c288() -> ()  [unwired: 1 in, 1 out]
        n158 = local read "Theta Actual (rad)"() -> (w339:dbl)
        n159 = Increment(x=w349) -> (x+1=w345:dbl)
        n160 = local read "Max speed"() -> (w335:dbl)
        n161 = shared-variable ".\\Robot Data Variables.lvlib\\Robot XY Position (m)"() -> (w326:dbl[])  [unwired: 1 in, 1 out]
        n162 = Divide(x=w335, y=0.01) -> (x/y=w337:dbl)
        n163 = Subtract(x=w339, y=w348) -> (x-y=w346:dbl)
        n164 = Absolute Value(x=w346) -> (abs(x)=w343:dbl)
        n165 = Max & Min(x=w345, y=w337) -> (min(x,y)=w334:dbl)  [unwired: 1 out]
        n166 = expression code="(x/pi)*180.0" "radians to degrees"(w343) -> (w342:dbl)
        n167 = call "VFH Wrapper (SubVI).vi"("Theta Actual (rad)"=w339, "Goal Position (m)"="Goal Position (m)", "Current Position (m)"=w326) -> ("Error Out"=w351:errorcluster, "Min Speed (m/s)"=→"Min speed":dbl, "Max Speed (m/s)"=→"Max speed":dbl, "chosen heading (rad)"=→"chosen heading (rad)":dbl)  [unwired: 5 in]
        n168 = Divide(x=w342, y=60.0) -> (x/y=w330:dbl)
        n169 = Max & Min(x=w331, y=w330) -> (min(x,y)=w329:dbl)  [unwired: 1 out]
        n170 = Subtract(x=w331, y=w329) -> (x-y=w332:dbl)
        n171 = local read "Min speed"() -> (w327:dbl)
        n172 = Multiply(x=w332, y=w334) -> (x*y=w344:dbl)
        n173 = Multiply(x=w344, y=0.01) -> (x*y=w341:dbl)
        n174 = Add(x=w341, y=w327) -> (x+y=→"speed setpoint (m/s)":dbl)
        n175 = local read "Stop"() -> (w353:bool)
        n176 = node-c288() -> ()  [unwired: 1 in, 1 out]
      }
      n177 = call "VFH Visualization.vi"() -> ()  [unwired: 3 in]
      n178 = node-c288(w23) -> ()  [unwired: 1 out]
      n179 = node-c288(w39) -> (w36:errorcluster)
      n180 = Merge Errors(w36, w35, w25, w21, w14) -> (w37:errorcluster)
    }
    frame #2 {
      # "Close"
      n181 = Merge Errors(w810) -> (w809:errorcluster)
      n182 = VISA Close(VISA resource name=w811) -> ()  [unwired: 1 in, 1 out]
      n183 = call <vilib>:"Reset myRIO.vi"("error in (no error)"=w809) -> ("error out"=→"Error Out":errorcluster)  [unwired: 10 in]
    }
  }
